vi "Runner.FilterExcludeVIList.vi"(10 "Paths":path[](array[path]), 11 "Test Runner":refnum<class "Test Runner.lvclass">) -> (2 "Filtered Paths":path[](array[path]), 3 "Test Runner":refnum<class "Test Runner.lvclass">)   [LabVIEW 2013, in "Caraya.lvlib" / "Test Runner.lvclass"]
uses:
  Test Runner/Test Runner.lvclass
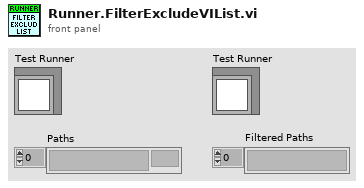
[diagram p1: front panel]
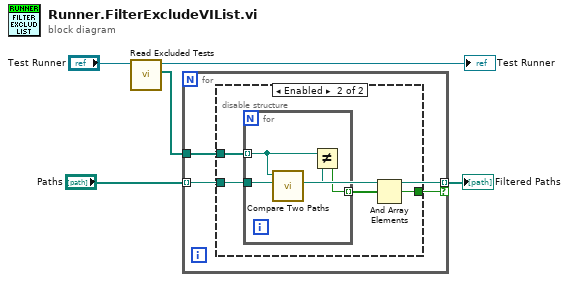
[diagram p0: block diagram]
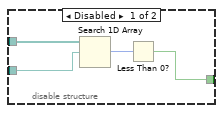
[diagram p2: hidden frame]
diagram:
  n1 = call "Read Excluded Tests.vi"("Test Runner in"="Test Runner") -> ("Excluded Tests"=w5:path[], "Test Runner out"=→"Test Runner":refnum<class "Test Runner.lvclass">)  [unwired: 8 in, 1 out]
  n2 = for {
    tunnel: "Paths" -> [w8] mode=indexing
    tunnel: [w8] -> w4 mode=indexing if=w7
    tunnel: w5 -> [w6]
    n3 = disable-structure shown="Enabled" {
      disable-tunnel: w8 -> [w12 w15]
      disable-tunnel: [w11 w13] -> w7
      disable-tunnel: w6 -> [w9 w16]
      frame Disabled {
        n4 = Search 1D Array(1D array=w9, element=w12) -> (index of element=w10:i32)  [unwired: 1 in]
        n5 = Less Than 0?(x=w10) -> (x < 0?=w11:bool)
      }
      frame Enabled {
        n6 = for {
          tunnel: w16 -> [w18] mode=indexing
          tunnel: w15 -> [w20]
          tunnel: [w17] -> w14 mode=indexing
          n7 = call <vilib>:"Compare Two Paths.vi"("Path 2"=w20, "Path 1"=w18) -> ("Common Path"=w19:path)  [unwired: 6 in, 3 out]
          n8 = Not Equal?(x=w18, y=w19) -> (x != y?=w17:bool)
        }
        n9 = And Array Elements(Boolean array=w14) -> (logical AND=w13:bool)
      }
    }
  }
  "Filtered Paths" <- w4
